vi "Actor Core.vi"(8 "error in":errorcluster, 11 "Host MSS Test Actor in":refnum<class "Host MSS Test Actor.lvclass">) -> (0 "error out":errorcluster, 3 "Actor out":refnum<class "Actor.lvclass">)   [LabVIEW 2023, in "Host MSS Test Actor.lvlib" / "Host MSS Test Actor.lvclass"]
doc: "(<B>Filename</B>: Actor Framework.lvlib:Actor.lvclass:Actor Core.vi)\n\nReceives messages to the actor, reacts to them, and initiates any error handling that may shut the actor down.\n\nDescendant classes may override this VI to append parallel tasks for the actor to complete while it handles messages. Overrides use the Call Parent Class Method node."
uses:
  Host MSS Test Actor.lvclass
  C:/Program Files/National Instruments/LabVIEW 2023/vi.lib/ActorFramework/Actor/Actor.lvclass
  <vilib>/ActorFramework/Actor/Actor.lvclass
  <vilib>/ni/Actors/Network Endpoint Actors/Notifying Nested Endpoint/Notifying Nested Endpoint.lvclass
  C:/Program Files/National Instruments/LabVIEW 2023/vi.lib/ni/Actors/Network Endpoint Actors/Network Endpoint/Network Endpoint/Network Endpoint.lvclass
  <vilib>/ActorFramework/Actor/Actor.lvclass/Actor.ctl
  <vilib>/ActorFramework/Message Enqueuer/Message Enqueuer.lvclass/Message Enqueuer.ctl
  Host MSS Test Actor.lvclass/Host MSS Test Actor.ctl
  <vilib>/ni/Actors/Network Endpoint Actors/Network Endpoint/Network Endpoint/Network Endpoint.lvclass/Network Endpoint.ctl
  <vilib>/ActorFramework/Message Enqueuer/Init from Existing Queue.vi
  <vilib>/ActorFramework/Message Enqueuer/Enqueue.vi
  Host MSS Test Actor Messages/Init Instrs Msg/Init Instrs Msg.lvclass
  C:/Program Files/National Instruments/LabVIEW 2023/vi.lib/ActorFramework/Message/Message.lvclass
  <vilib>/ActorFramework/Stop Msg/Stop Msg.lvclass
  <vilib>/Utility/LVClass/Get LV Class Name.vi
  <resource>/AFDebug/Generate Trace for Message.vi
  <vilib>/ActorFramework/Message Priority Queue/Priority Enqueue.vi
  <vilib>/ActorFramework/Message Enqueuer/Message Enqueuer.lvclass
  <vilib>/ni/Actors/Network Endpoint Actors/Network Endpoint/Network Endpoint/Network Endpoint.lvclass
  D:/git/HAL/HAL GOOP4/Host Measure and Stimulus Subsystems/Tests/Host MSS Test Actor/Host MSS Test Actor/Host MSS Test Actor.lvclass
  C:/Program Files/National Instruments/LabVIEW 2023/vi.lib/ni/Actors/Network Endpoint Actors/Nested Endpoint Caller/Nested Endpoint Caller/Nested Endpoint Caller.lvclass
  C:/Program Files/National Instruments/LabVIEW 2023/vi.lib/ni/Actors/Network Endpoint Actors/Nested Endpoint/Nested Endpoint/Nested Endpoint.lvclass
  C:/Program Files/National Instruments/LabVIEW 2023/vi.lib/ni/Actors/Network Endpoint Actors/Notifying Nested Endpoint/Notifying Nested Endpoint.lvclass
panel:
  in  "Kill cRIO Button":bool
  in  "Init Instrs Button":bool
  out "Connected":bool
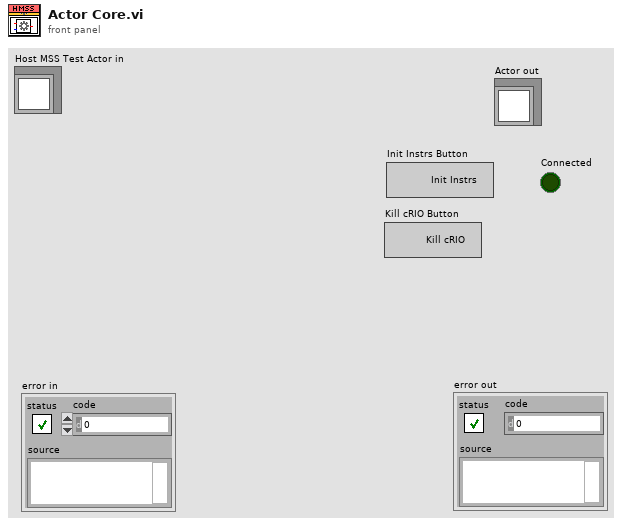
[diagram p1: front panel]
types:
  T1 = cluster{"Stop":refnum<user-event>, "Connected":refnum<user-event>}
  T2 = map{string, refnum<class "Message Enqueuer.lvclass">}
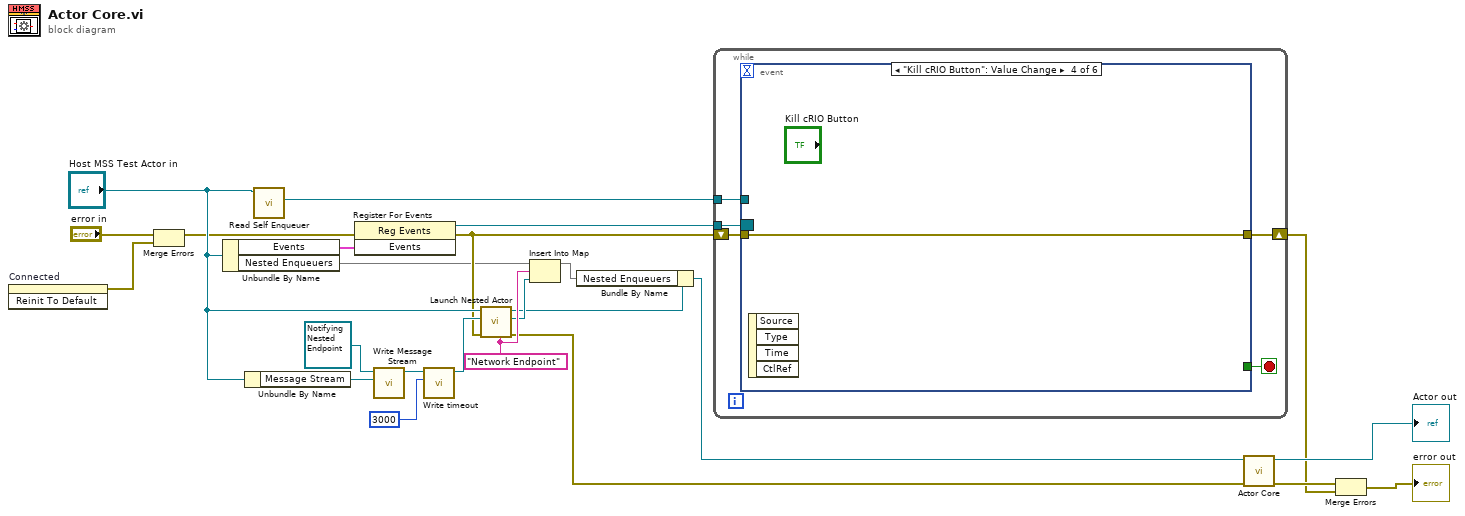
[diagram p0: block diagram]
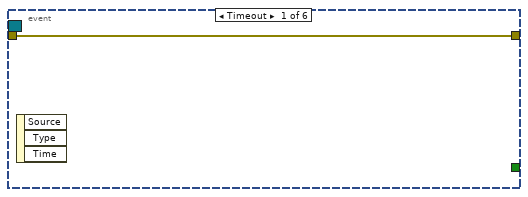
[diagram p2: hidden frame]
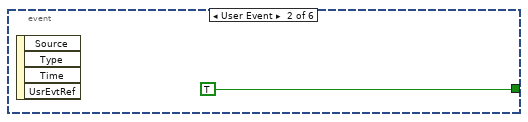
[diagram p3: hidden frame]
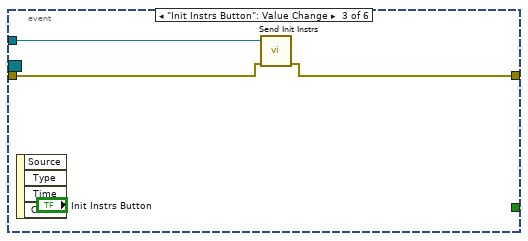
[diagram p4: hidden frame]
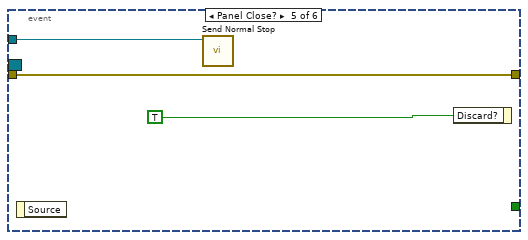
[diagram p5: hidden frame]
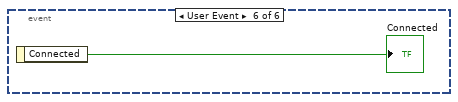
[diagram p6: hidden frame]
diagram:
  w11 = "Network Endpoint" ("Debug Alias")
  n1 = invoke on="Connected" class="Bool (strict)" method="Reinit To Default"() -> (error out=w1:errorcluster)  [unwired: 3 in, 2 out]
  n2 = Merge Errors("error in", w1) -> (w2:errorcluster)
  n3 = Unbundle By Name("Host MSS Test Actor in") -> ("Events"=w22:T1, "Nested Enqueuers"=w3:T2)
  n4 = Unbundle By Name("Host MSS Test Actor in") -> ("Message Stream"=w15:refnum<class "Message Stream.lvclass">)
  n5 = call <vilib>:"Read Self Enqueuer.vi"("Actor"="Host MSS Test Actor in") -> ("Self Enqueuer"=w14:refnum<class "Message Enqueuer.lvclass">)  [unwired: 10 in]
  n6 = register-events(error in=w2, w22) -> (reference out=w21:refnum<event-registration>, error out=w7:errorcluster)  [unwired: 1 in]
  n7 = call <vilib>:"Write Message Stream.vi"("Message Stream"=w15, "Network Endpoint in"=refnum<class "Notifying Nested Endpoint.lvclass"> refnum ("Notifying Nested Endpoint.lvclass")) -> ("Network Endpoint out"=w17:refnum<class "Notifying Nested Endpoint.lvclass">)  [unwired: 9 in]
  n8 = call <vilib>:"Write timeout.vi"("timeout"=3000, "Network Endpoint in"=w17) -> ("Network Endpoint out"=w13:refnum<class "Notifying Nested Endpoint.lvclass">)  [unwired: 9 in]
  n9 = call <vilib>:"Launch Nested Actor.vi"("Debug Alias"=w11, "error in (no error)"=w7, "Nested Actor"=w13, "Caller Actor in"="Host MSS Test Actor in") -> ("error out"=w6:errorcluster, "Nested Actor's Enqueuer"=w10:refnum<class "Message Enqueuer.lvclass">, "Caller Actor out"=w9:refnum<class "Host MSS Test Actor.lvclass">)  [unwired: 5 in]
  n10 = Insert Into Map(map in=w3, key=w11, value=w10) -> (map out=w4:T2)  [unwired: 2 out]
  n11 = Bundle By Name(cluster=w9, "Nested Enqueuers"=w4) -> (w5:refnum<class "Host MSS Test Actor.lvclass">)
  n12 = while {
    tunnel: w21 -> [w29]
    shift-right: [w27] -> w19
    shift-left: w7 -> [w28]
    tunnel: w14 -> [w25]
    stop <- w26 stop-if-true
    n13 = event shown="[3] \"Kill cRIO Button\": Value Change" {
      selector: w29 -> [_ _ _ _ _ _]
      dyn-events: _ -> [_ _ _ _ _ _]
      timeout: _ -> [_ _ _ _ _ _]
      tunnel: w28 -> [w30 _ w33 w35 w36 _]
      tunnel: [w30 _ w32 w35 w36 _] -> w27
      tunnel: [_ TRUE _ _ _ _] -> w26
      tunnel: w25 -> [_ _ w34 _ w37 _]
      event Timeout {
        n14 = event-data() -> ()  [unwired: 1 in, 3 out]
      }
      event User Event {
        n15 = event-data() -> ()  [unwired: 1 in, 4 out]
      }
      event "Init Instrs Button": Value Change {
        n16 = event-data() -> ()  [unwired: 1 in, 4 out]
        n17 = call "Send Init Instrs.vi"("error in (no error)"=w33, "Message Enqueuer"=w34) -> ("error out"=w32:errorcluster)  [unwired: 8 in, 1 out]
      }
      event "Kill cRIO Button": Value Change {
        n18 = event-data() -> ()  [unwired: 1 in, 4 out]
      }
      event Panel Close? {
        n19 = event-data() -> ()  [unwired: 1 in, 1 out]
        n20 = call <vilib>:"Send Normal Stop.vi"("Message Enqueuer"=w37) -> ()  [unwired: 10 in, 1 out]
        n21 = event-data("Discard?"=TRUE) -> ()  [unwired: 1 in, 1 out]
      }
      event User Event {
        n22 = event-data() -> ("Connected"=→"Connected":bool)  [unwired: 1 in]
      }
    }
  }
  n23 = call-parent "Actor Core.vi"("error in"=w6, "Actor in"=w5) -> ("error out"=w24:errorcluster, "Actor out"=→"Actor out":refnum<class "Actor.lvclass">)  [unwired: 8 in]
  n24 = Merge Errors(w24, w19) -> (→"error out":errorcluster)
